vi "IP9258_POWER_Off_WebSwitch.vi"() -> ()   [LabVIEW 2011]
doc: "Example of using standard HTTP protocol for recieving a web site (the HTML source)\n\n\nThis example uses the GET command. For general information about the HTTP protocol and other commands go to\nhttp://www.w3.org/Protocols\n\n\nBjornar Svingen\nbjornar.svingen@sintef.no bjornar.svingen@ktv.no"
uses:
  <vilib>/addons/internet/telnet/telnet.llb/Telnet Session.ctl
  <vilib>/addons/internet/NI_InternetTK_Core_VIs.lvlib
panel:
  out "log2":string
  out "telnet connection":T1
  out "log1":string
  out "DebugView":string
  out "Begin Time":u32
  # "2014-8-25"
  # "IP9258 Power Off"
  # "All 4 Ports Off"
  # "本程式是Telnet方式來控制IP9258\n1.Windows 需開啟Telnet 服務( Need eable Telnet Client Service)\n2.IP_POWER_WEB_SWITCH_IP=?;       /* need define it /\n3.IP9258_ACCOUNT_PASSWORD=?; /* need define it */"
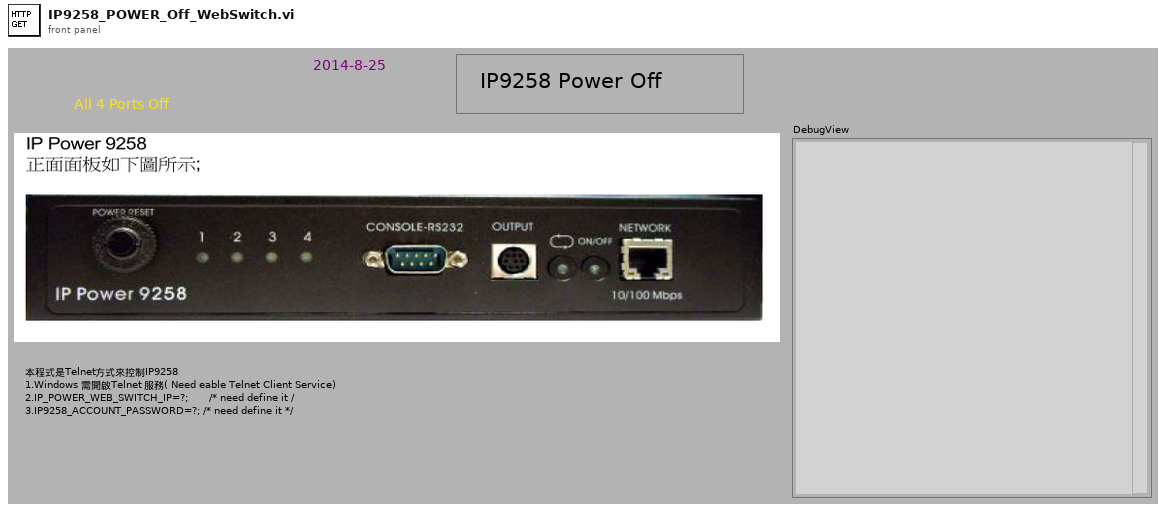
[diagram p1: front panel]
types:
  T1 = typedef "Telnet Session.ctl" = refnum<k1>
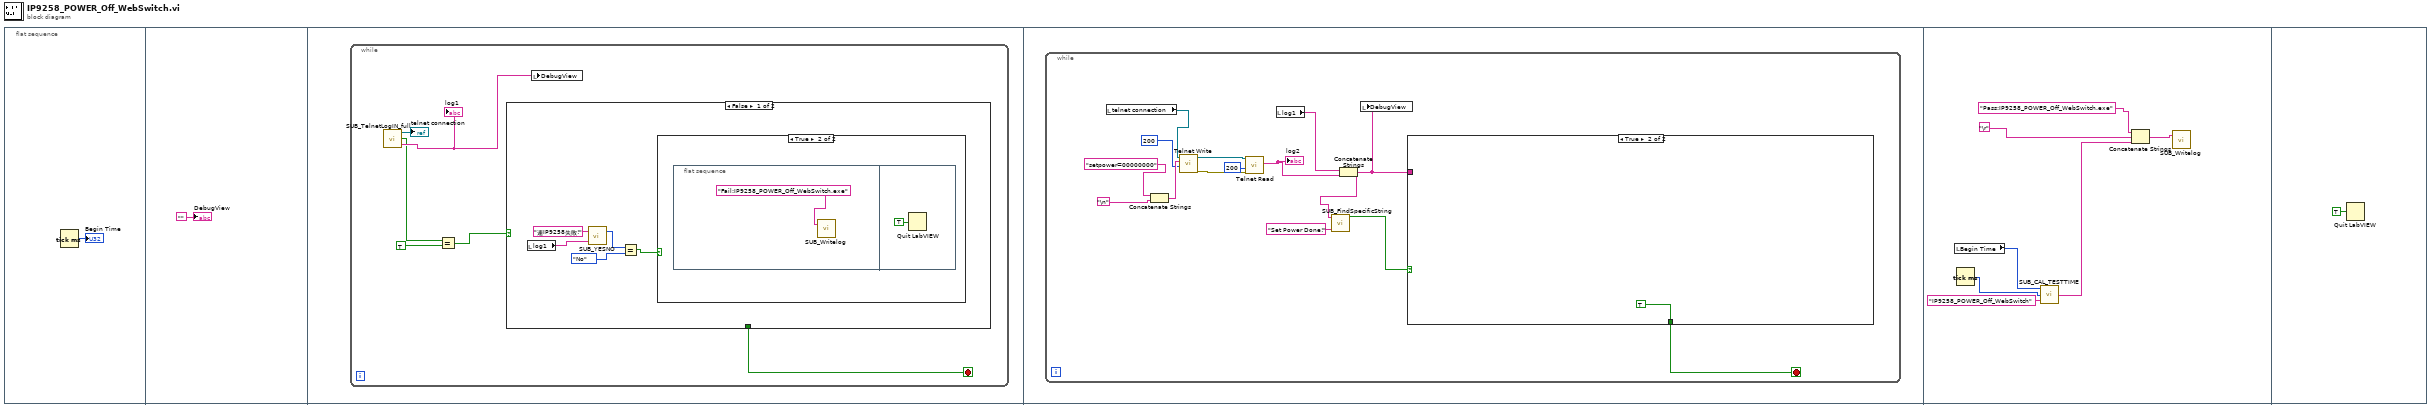
[diagram p0: block diagram]
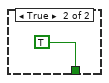
[diagram p3: hidden frame]
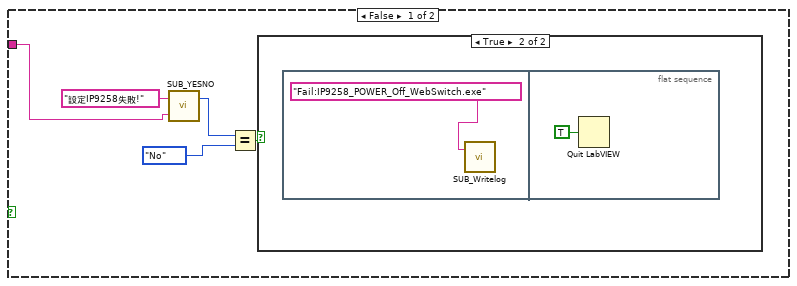
[diagram p4: hidden frame]
diagram:
  n1 = flat-sequence {
    frame #0 {
      n2 = Tick Count (ms)() -> (millisecond timer value=→"Begin Time":u32)
    }
    frame #1 {
      "DebugView" <- ""
    }
    frame #2 {
      n3 = while {
        stop <- w4 stop-if-true
        n4 = call "SUB_TelnetLogIN_full.vi"() -> ("telnet connection"=→"telnet connection":T1, "Pass ?"=w7:bool, "data out"=w8:string)  [unwired: 2 in]
        "log1" <- w8
        n5 = Equal?(x=w7, y=TRUE) -> (x = y?=w5:bool)
        n6 = case shown="False" w5 {
          tunnel: [_ TRUE] -> w4
          frame False {
            n7 = local read "log1"() -> (w13:string)
            n8 = call "SUB_YESNO.vi"("Debug View"=w13, "Status"="連IP9258失敗!") -> ("yes/no"=w11:enum32{"No Selection", "Yes", "No", "None"})  [unwired: 1 in]
            n9 = Equal?(x=w11, y=enum32{"No Selection", "Yes", "No", "None"}."No") -> (x = y?=w9:bool)
            n10 = case shown="True" w9 {
              frame False {
              }
              frame True {
                n11 = flat-sequence {
                  frame #0 {
                    n12 = call "SUB_Writelog.vi"("Pass/Fail"="Fail:IP9258_POWER_Off_WebSwitch.exe") -> ()  [unwired: 2 in]
                  }
                  frame #1 {
                    n13 = Quit LabVIEW(quit? (T)=TRUE) -> ()
                  }
                }
              }
            }
          }
          frame True {
          }
        }
        n14 = local write "DebugView"(w8) -> ()
      }
    }
    frame #3 {
      n15 = while {
        stop <- w18 stop-if-true
        n16 = local read "telnet connection"() -> (w30:T1)
        n17 = Concatenate Strings("setpower=00000000" ("data in"), "\n") -> (w24:string)
        n18 = call <vilib>:"Telnet Write.vi"("timeout ms (25000)"=200, "data in"=w24, "telnet connection"=w30) -> ("error out"=w28:errorcluster, "telnet connection out"=w29:T1)  [unwired: 4 in, 1 out]
        n19 = call <vilib>:"Telnet Read.vi"("error in (no error)"=w28, "timeout ms (25000)"=200, "telnet connection"=w29) -> ("data out"=w26:string)  [unwired: 4 in, 2 out]
        "log2" <- w26
        n20 = local read "log1"() -> (w27:string)
        n21 = Concatenate Strings(w27, w26) -> (w17:string)
        n22 = call "SUB_FindSpecificString.vi"("Find this String"="Set Power Done!", "String data"=w17) -> ("Found"=w19:bool)  [unwired: 2 in, 1 out]
        n23 = local write "DebugView"(w17) -> ()
        n24 = case shown="True" w19 {
          tunnel: [_ TRUE] -> w18
          tunnel: w17 -> [w34 _]
          frame False {
            n25 = call "SUB_YESNO.vi"("Debug View"=w34, "Status"="設定IP9258失敗!") -> ("yes/no"=w32:enum32{"No Selection", "Yes", "No", "None"})  [unwired: 1 in]
            n26 = Equal?(x=w32, y=enum32{"No Selection", "Yes", "No", "None"}."No") -> (x = y?=w31:bool)
            n27 = case shown="True" w31 {
              frame False {
              }
              frame True {
                n28 = flat-sequence {
                  frame #0 {
                    n29 = call "SUB_Writelog.vi"("Pass/Fail"="Fail:IP9258_POWER_Off_WebSwitch.exe") -> ()  [unwired: 2 in]
                  }
                  frame #1 {
                    n30 = Quit LabVIEW(quit? (T)=TRUE) -> ()
                  }
                }
              }
            }
          }
          frame True {
          }
        }
      }
    }
    frame #4 {
      n31 = local read "Begin Time"() -> (w45:u32)
      n32 = Tick Count (ms)() -> (millisecond timer value=w44:u32)
      n33 = call "SUB_CAL_TESTTIME.vi"("Test Item name"="IP9258_POWER_Off_WebSwitch", "Stop tick time"=w44, "Start tick time"=w45) -> ("Test Time output"=w40:string)  [unwired: 2 in]
      n34 = Concatenate Strings("Pass:IP9258_POWER_Off_WebSwitch.exe", "\r", w40) -> (w39:string)
      n35 = call "SUB_Writelog.vi"("Pass/Fail"=w39) -> ()  [unwired: 2 in]
    }
    frame #5 {
      n36 = Quit LabVIEW(quit? (T)=TRUE) -> ()
    }
  }
